vi "5790A ac meas.vi"(6 "error in":errorcluster, 9 "5790A":refnum<visa-resource-name>) -> (0 "error out":errorcluster, 1 "Frequency":dbl, 2 "Voltage":dbl, 3 "Session Out":refnum<visa-resource-name>, 4 "code":dbl, 5 "read buffer":string)   [LabVIEW 2020]
panel:
  out "error out 2":errorcluster
  out "Numeric":i32
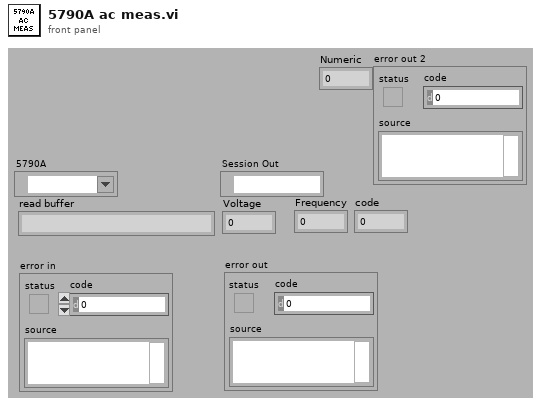
[diagram p1: front panel]
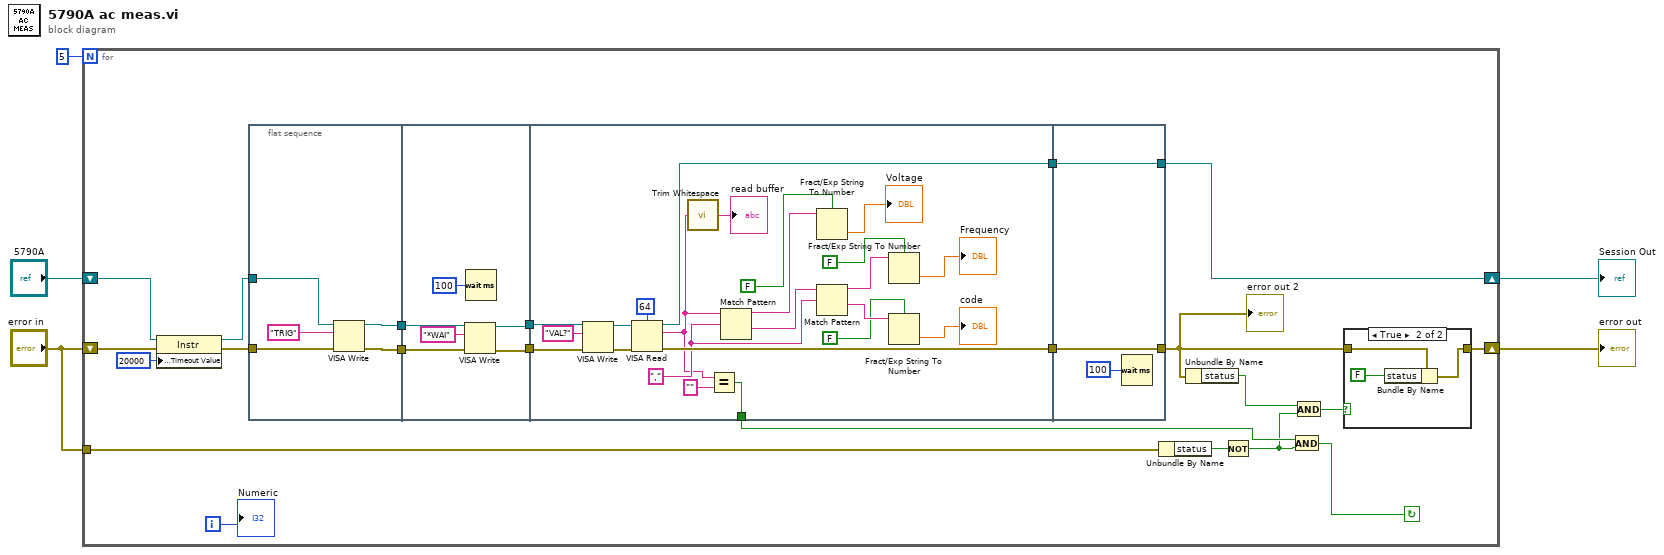
[diagram p0: block diagram]
diagram:
  n1 = for {
    N: 5 -> [_]
    shift-right: [w21] -> w5
    shift-left: "5790A" -> [w12]
    shift-right: [w17] -> w4
    shift-left: "error in" -> [w14]
    tunnel: "error in" -> [w20]
    i -> [w16]
    stop <- w18 continue-if-true
    n2 = property class="Instr"(reference=w12, error in=w14, "General Settings:Timeout Value"=u32 20000) -> (reference out=w11:refnum<visa-resource-name>, error out=w13:errorcluster)
    n3 = flat-sequence {
      tunnel: [w33] -> w27
      tunnel: [w32] -> w26
      tunnel: w11 -> [w36]
      tunnel: w13 -> [w35]
      tunnel: w27 -> [w41]
      tunnel: [w40] -> w25
      tunnel: w26 -> [w38]
      tunnel: [w39] -> w24
      tunnel: w25 -> [w47]
      tunnel: [w65] -> w23
      tunnel: w24 -> [w46]
      tunnel: [w64] -> w22
      tunnel: [w49] -> w10
      tunnel: w23 -> [w68]
      tunnel: w22 -> [w67]
      tunnel: [w68] -> w9
      tunnel: [w67] -> w21
      frame #0 {
        n4 = VISA Write(VISA resource name=w36, write buffer="TRIG", error in (no error)=w35) -> (VISA resource name out=w32:refnum<visa-resource-name>, error out=w33:errorcluster)  [unwired: 1 out]
      }
      frame #1 {
        n5 = VISA Write(VISA resource name=w38, write buffer="*WAI", error in (no error)=w41) -> (VISA resource name out=w39:refnum<visa-resource-name>, error out=w40:errorcluster)  [unwired: 1 out]
        n6 = Wait (ms)(milliseconds to wait=u32 100) -> ()  [unwired: 1 out]
      }
      frame #2 {
        w59 = "," ("regular expression")
        n7 = VISA Write(VISA resource name=w46, write buffer="VAL?", error in (no error)=w47) -> (VISA resource name out=w45:refnum<visa-resource-name>, error out=w48:errorcluster)  [unwired: 1 out]
        n8 = VISA Read(VISA resource name=w45, byte count=u32 64, error in (no error)=w48) -> (VISA resource name out=w64:refnum<visa-resource-name>, read buffer=w51:string, error out=w65:errorcluster)  [unwired: 1 out]
        n9 = call <vilib>:"Trim Whitespace.vi"("string"=w51) -> ("trimmed string"=→"read buffer":string)  [unwired: 1 in]
        n10 = Equal?(x=w51, y="") -> (x = y?=w49:bool)
        n11 = Match Pattern(string=w51, regular expression=w59) -> (before substring=w61:string, after substring=w60:string)  [unwired: 1 in, 2 out]
        n12 = Fract/Exp String To Number(use system decimal point (T)=FALSE, string=w61) -> (number=→"Voltage":dbl)  [unwired: 2 in, 1 out]
        n13 = Match Pattern(string=w60, regular expression=w59) -> (before substring=w57:string, after substring=w58:string)  [unwired: 1 in, 2 out]
        n14 = Fract/Exp String To Number(use system decimal point (T)=FALSE, string=w57) -> (number=→"Frequency":dbl)  [unwired: 2 in, 1 out]
        n15 = Fract/Exp String To Number(use system decimal point (T)=FALSE, string=w58) -> (number=→"code":dbl)  [unwired: 2 in, 1 out]
      }
      frame #3 {
        n16 = Wait (ms)(milliseconds to wait=u32 100 ("millisecond multiple")) -> ()  [unwired: 1 out]
      }
    }
    n17 = Unbundle By Name(w20) -> ("status"=w19:bool)
    n18 = Unbundle By Name(w9) -> ("status"=w8:bool)
    n19 = Not(x=w19) -> (.not. x?=w7:bool)
    n20 = And(x=w10, y=w7) -> (x .and. y?=w18:bool)
    n21 = And(x=w8, y=w7) -> (x .and. y?=w6:bool)
    n22 = case shown="True" w6 {
      tunnel: [w28 w30] -> w17
      tunnel: w9 -> [w28 w31]
      frame False {
      }
      frame True {
        n23 = Bundle By Name(cluster=w31, "status"=FALSE) -> (w30:errorcluster)
      }
    }
    "Numeric" <- w16
    "error out 2" <- w9
  }
  "Session Out" <- w5
  "error out" <- w4
